vi "getDevices.vi"(8 "error in (no error)":errorcluster, 11 "ACNET Devices in":refnum<class "ACNET Devices.lvclass">) -> (0 "error out":errorcluster, 2 "Devices":refnum<class "ACNET Device.lvclass">[](array[class]), 3 "ACNET Devices out":refnum<class "ACNET Devices.lvclass">)   [LabVIEW 2013, in "ACNET Monitor.lvlib" / "ACNET Devices.lvclass"]
uses:
  ACNET Devices.lvclass
  ACNET Device.lvclass
  ACNET Devices.lvclass/ACNET Devices.ctl
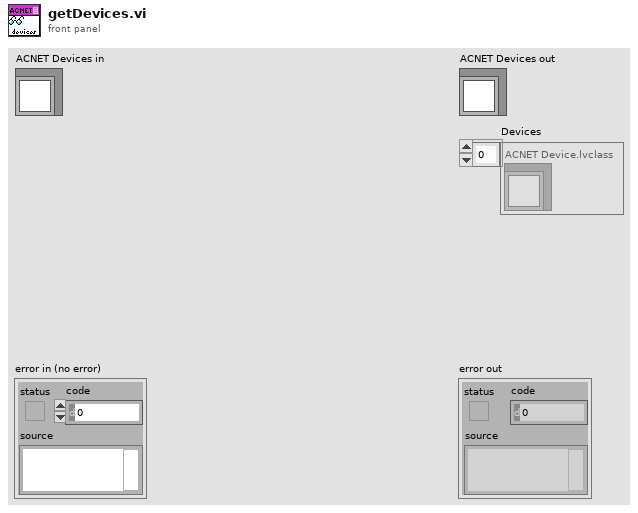
[diagram p1: front panel]
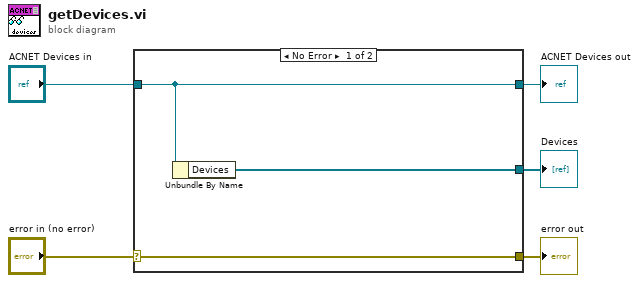
[diagram p0: block diagram]
diagram:
  n1 = case shown="No Error" "error in (no error)" {
    selector: "error in (no error)" -> [w8 w9]
    tunnel: [w8 w9] -> w4
    tunnel: [w7 w10] -> w2
    tunnel: "ACNET Devices in" -> [w7 w10]
    tunnel: [w6 _] -> w1
    frame No Error {
      n2 = Unbundle By Name(w7) -> ("Devices"=w6:refnum<class "ACNET Device.lvclass">[])
    }
    frame Error {
    }
  }
  "error out" <- w4
  "ACNET Devices out" <- w2
  "Devices" <- w1
